vi "bufferBoard.vi"(3 "?":i32) -> (20 "silica":bool, 21 "peak":bool, 22 "qdc1":bool, 23 "qdc2":bool, 24 "tdc1":bool, 25 "qdc3":bool, 26 "tdc2":bool, 27 "null":bool)   [LabVIEW 2014]
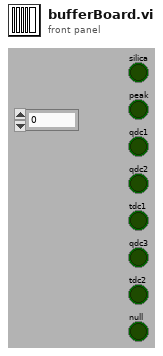
[diagram p1: front panel]
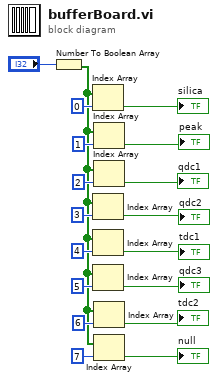
[diagram p0: block diagram]
diagram:
  n1 = Number To Boolean Array(number="?") -> (Boolean array=w10:bool[])
  n2 = Index Array(array=w10, index=0) -> (element=→"silica":bool)
  n3 = Index Array(array=w10, index=3) -> (element=→"qdc2":bool)
  n4 = Index Array(array=w10, index=4) -> (element=→"tdc1":bool)
  n5 = Index Array(array=w10, index=5) -> (element=→"qdc3":bool)
  n6 = Index Array(array=w10, index=1) -> (element=→"peak":bool)
  n7 = Index Array(array=w10, index=2) -> (element=→"qdc1":bool)
  n8 = Index Array(array=w10, index=6) -> (element=→"tdc2":bool)
  n9 = Index Array(array=w10, index=7) -> (element=→"null":bool)
